vi "Test UNSUBSCRIBE packet.vi"() -> ()   [LabVIEW 2013]
uses:
  source/Control Packets/UNSUBSCRIBE/UNSUBSCRIBE.lvclass
  source/Control Packets/ControlPacket/ControlPacket.lvclass/ControlPacket.ctl
  source/Control Packets/ControlPacket/ControlPacket.lvclass
panel:
  out "Subscription Payload":bool
  out "Packet ID":u16 format="%04x"
  out "error out":errorcluster
  out "Packet Identifier":bool
  out "Packet type":bool
  out "All packets consumed":bool
  out "Complete Packet":bool
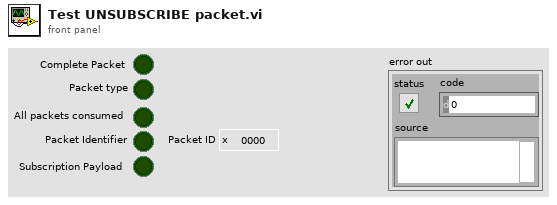
[diagram p1: front panel]
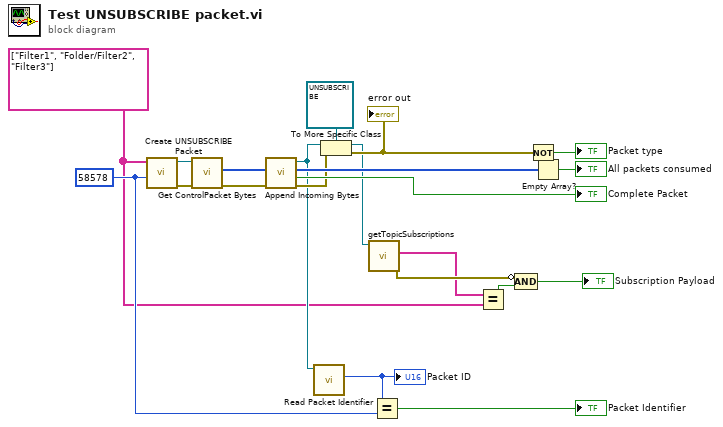
[diagram p0: block diagram]
diagram:
  w4 = string[] ["Filter1", "Folder/Filter2", "Filter3"] ("Topic Subscriptions")
  w7 = u16 58578 ("Packet ID")
  n1 = call "Create UNSUBSCRIBE Packet.vi"("Packet ID"=w7, "Topic Subscriptions"=w4) -> ("error out"=w6:errorcluster, "UNSUBSCRIBE out"=w5:refnum<class "UNSUBSCRIBE.lvclass">)  [unwired: 8 in]
  n2 = call "Get ControlPacket Bytes.vi"("error in (no error)"=w6, "ControlPacket"=w5) -> ("error out"=w16:errorcluster, "Bytes Stream"=w21:u8[])  [unwired: 7 in, 1 out]
  n3 = call "Append Incoming Bytes.vi"("error in (no error)"=w16, "Incoming Packets"=w21) -> ("error out"=w15:errorcluster, "Complete Packet"=→"Complete Packet":bool, "Remaining Packets"=w19:u8[], "ControlPacket"=w12:refnum<class "ControlPacket.lvclass">)  [unwired: 6 in]
  n4 = call "Read Packet Identifier.vi"("ControlPacket in"=w12) -> ("Packet Identifier"=w14:u16)  [unwired: 9 in, 1 out]
  "Packet ID" <- w14
  n5 = To More Specific Class(target class=refnum<class "UNSUBSCRIBE.lvclass"> refnum ("UNSUBSCRIBE.lvclass"), reference=w12, error in=w15) -> (specific class reference=w3:refnum<class "UNSUBSCRIBE.lvclass">, error out=w11:errorcluster)
  "error out" <- w11
  n6 = call "getTopicSubscriptions.vi"("UNSUBSCRIBE in"=w3) -> ("error out"=w2:errorcluster, "Topic Subscriptions"=w1:string[])  [unwired: 8 in, 1 out]
  n7 = Equal?(x=w14, y=w7) -> (x = y?=→"Packet Identifier":bool)
  n8 = Equal?(x=w1, y=w4) -> (x = y?=w10:bool)
  n9 = Compound Arithmetic op=AND(invert w2, w10) -> (→"Subscription Payload":bool)
  n10 = Not(x=w11) -> (.not. x?=→"Packet type":bool)
  n11 = Empty Array?(array=w19) -> (empty?=→"All packets consumed":bool)
